vi "test_Delete Instrument Addon.vi"(8 "error in (no error)":errorcluster, 11 "TestCase in":refnum<class "Instrument Addon Scripting API Custom Device Unit Tests.lvclass">) -> (0 "error out":errorcluster, 3 "TestCase out":refnum<class "Instrument Addon Scripting API Custom Device Unit Tests.lvclass">)   [LabVIEW 2021, in "Instrument Addon Scripting API Custom Device Unit Tests.lvclass"]
uses:
  Instrument Addon Scripting API Custom Device Unit Tests.lvclass
  Instrument Addon Scripting API Custom Device Unit Tests.lvclass/Instrument Addon Scripting API Custom Device Unit Tests.ctl
  <vilib>/addons/_JKI Toolkits/VI Tester/TestCase.llb/TestCase.lvclass
  Addon/Addon Shared/SubVIs/Constants.vi
  Addon/Addon Shared/Instrument Addon Shared.lvlib
  NationalInstruments.VeriStand.SystemDefinitionAPI
  APIs/Scripting API/Instrument Addon Scripting API.lvlib
  <vilib>/NI VeriStand/Custom Device Tools/Custom Device Utility Library/Custom Device Utility Library.lvlib
  <vilib>/NI VeriStand/Custom Device Tools/Custom Device Utility Library/NI VeriStand - Search for Item by Name.vi
  C:/Program Files (x86)/National Instruments/LabVIEW 2020/vi.lib/addons/_JKI Toolkits/VI Tester/TestCase.llb/TestCase.lvclass
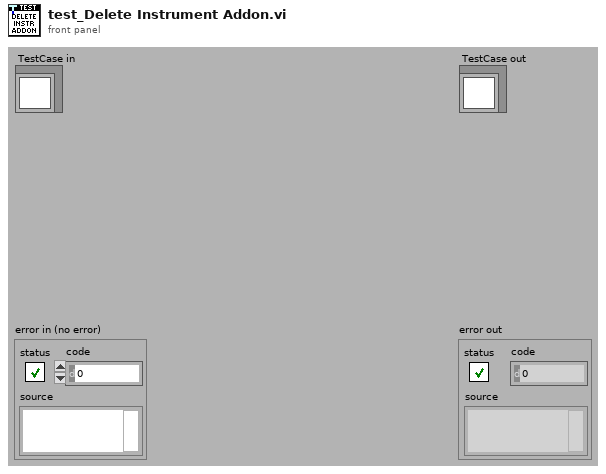
[diagram p1: front panel]
types:
  T1 = typedef "Custom Device API.lvlib/Custom Device Item Ref.ctl" = u64
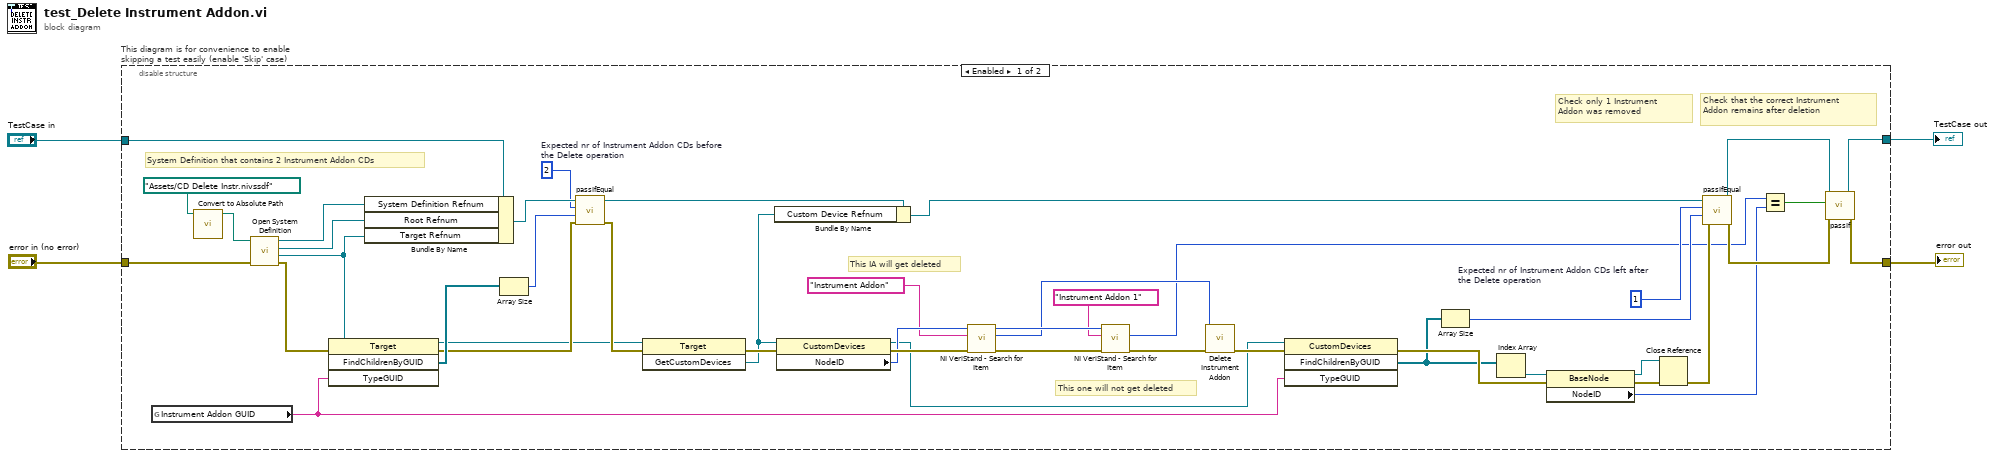
[diagram p0: block diagram]
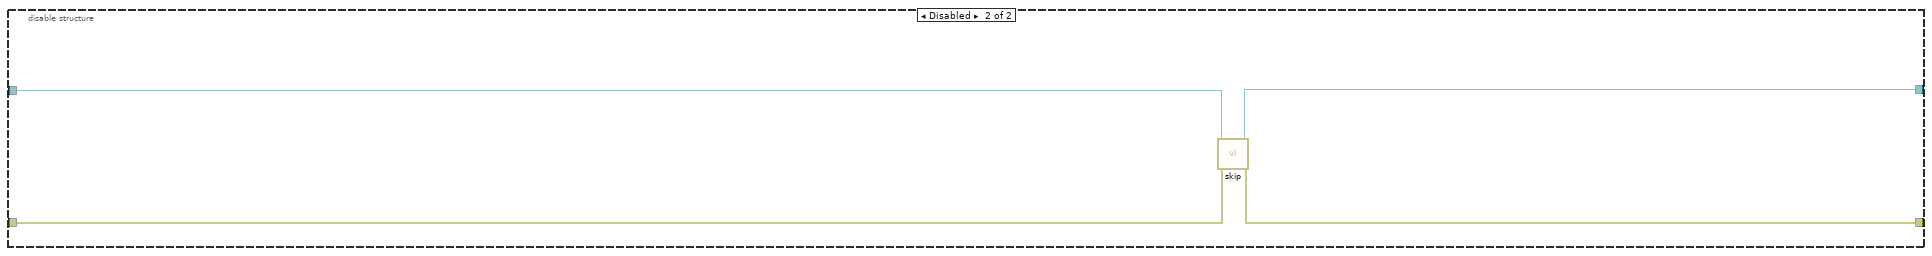
[diagram p2: hidden frame]
diagram:
  n1 = disable-structure "This diagram is for convenience to enable skipping a test easily (enable 'Skip' case)" shown="Enabled" {
    disable-tunnel: "TestCase in" -> [w36 w51]
    disable-tunnel: [w46 w50] -> w1
    disable-tunnel: [w47 w53] -> w3
    disable-tunnel: "error in (no error)" -> [w49 w52]
    frame Enabled {
      w24 = 2  # Expected nr of Instrument Addon CDs before the Delete operation
      w38 = 1  # Expected nr of Instrument Addon CDs left after the Delete operation
      # "This one will not get deleted"
      # "This IA will get deleted"
      # "Check only 1 Instrument Addon was removed"
      # "System Definition that contains 2 Instrument Addon CDs"
      # "Check that the correct Instrument Addon remains after deletion"
      n2 = global read "Constants.vi" "Instrument Addon GUID"() -> (w30:string)
      n3 = call "Convert to Absolute Path.vi"("System Definition File"=path "Assets/CD Delete Instr.nivssdf" ("SDF file")) -> ("Absolute Path"=w48:path)  [unwired: 10 in]
      n4 = call "Open System Definition.vi"("error in (no error)"=w49, "System Definition File"=w48) -> ("error out"=w29:errorcluster, "Target Refnum"=w22:refnum<k24>, "Root Refnum"=w34:refnum<k24>, "System Definition Refnum"=w35:refnum<k24>)  [unwired: 6 in]
      n5 = invoke class="Target" method="FindChildrenByGUID"(reference=w22, error in=w29, "TypeGUID"=w30) -> (reference out=w20:refnum<k24>, error out=w25:errorcluster, "FindChildrenByGUID"=w28:refnum<k24>[])  [unwired: 1 in, 1 out]
      n6 = Bundle By Name(cluster=w36, "System Definition Refnum"=w35, "Root Refnum"=w34, "Target Refnum"=w22) -> (w27:refnum<class "Instrument Addon Scripting API Custom Device Unit Tests.lvclass">)
      n7 = Array Size(array=w28) -> (size(s)=w23:i32)
      n8 = call-dynamic "passIfEqual.vi"("error in (no error)"=w25, "y"=w23, "x"=w24, "TestCase in"=w27) -> ("error out"=w21:errorcluster, "TestCase out"=w26:refnum<class "Instrument Addon Scripting API Custom Device Unit Tests.lvclass">)  [unwired: 6 in]
      n9 = invoke class="Target" method="GetCustomDevices"(reference=w20, error in=w21) -> (error out=w19:errorcluster, "GetCustomDevices"=w17:refnum<k24>)  [unwired: 1 in, 1 out]
      n10 = Bundle By Name(cluster=w26, "Custom Device Refnum"=w17) -> (w18:refnum<class "Instrument Addon Scripting API Custom Device Unit Tests.lvclass">)
      n11 = property class="CustomDevices"(reference=w17, error in=w19) -> (reference out=w8:refnum<k24>, error out=w16:errorcluster, "NodeID"=w15:u64)
      n12 = call-poly <vilib>:"NI VeriStand - Search for Item.vi"("error in"=w16, "Item Name"="Instrument Addon", "Section Ref in"=w15) -> ("error out"=w13:errorcluster, "Item Ref"=w10:T1, "Section Ref out"=w11:T1)  [unwired: 5 in, 1 out]
      n13 = call-poly <vilib>:"NI VeriStand - Search for Item.vi"("error in"=w13, "Item Name"="Instrument Addon 1", "Section Ref in"=w11) -> ("error out"=w12:errorcluster, "Item Ref"=w7:T1)  [unwired: 5 in, 2 out]
      n14 = call "Delete Instrument Addon.vi"("error in (no error)"=w12, "instrument addon refnum"=w10) -> ("error out"=w45:errorcluster)  [unwired: 9 in]
      n15 = invoke class="CustomDevices" method="FindChildrenByGUID"(reference=w8, error in=w45, "TypeGUID"=w30) -> (error out=w42:errorcluster, "FindChildrenByGUID"=w41:refnum<k24>[])  [unwired: 1 in, 2 out]
      n16 = Array Size(array=w41) -> (size(s)=w39:i32)
      n17 = Index Array(array=w41) -> (element=w43:refnum<k24>)  [unwired: 1 in]
      n18 = property class="BaseNode"(reference=w43, error in=w42) -> (reference out=w31:refnum<k24>, error out=w33:errorcluster, "NodeID"=w6:u64)
      n19 = Close Reference(reference=w31, error in (no error)=w33) -> (error out=w32:errorcluster)
      n20 = call-dynamic "passIfEqual.vi"("error in (no error)"=w32, "y"=w39, "x"=w38, "TestCase in"=w18) -> ("error out"=w40:errorcluster, "TestCase out"=w37:refnum<class "Instrument Addon Scripting API Custom Device Unit Tests.lvclass">)  [unwired: 6 in]
      n21 = Equal?(x=w7, y=w6) -> (x = y?=w5:bool)
      n22 = call-dynamic "passIf.vi"("error in (no error)"=w40, "pass"=w5, "TestCase in"=w37) -> ("error out"=w47:errorcluster, "TestCase out"=w46:refnum<class "Instrument Addon Scripting API Custom Device Unit Tests.lvclass">)  [unwired: 7 in]
    }
    frame Disabled {
      # "skip test result while test is under development"
      n23 = call <vilib>:"skip.vi"("error in (no error)"=w52, "TestCase in"=w51) -> ("error out"=w53:errorcluster, "TestCase out"=w50:refnum<class "Instrument Addon Scripting API Custom Device Unit Tests.lvclass">)  [unwired: 8 in]
    }
  }
  "error out" <- w3
  "TestCase out" <- w1
